vi "Subscribe to Request-Reply.vi"(8 "error in (no error)":errorcluster, 11 "Request-Reply Reference in":refnum<data-value>) -> (0 "error out":errorcluster, 3 "Request-Reply Reference out":refnum<data-value>)   [LabVIEW 2018, in "Scripting.lvlib"]
uses:
  Scripting.lvlib
  Actor/Stop.ctl
  Actor/Did Stop.ctl
  Actor/Actor.lvclass
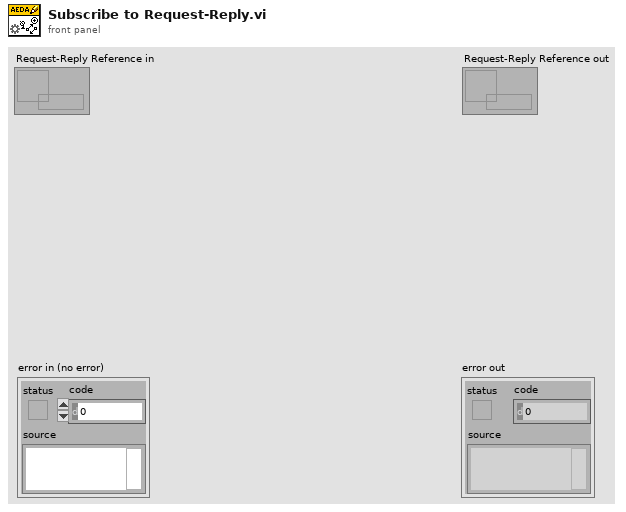
[diagram p1: front panel]
types:
  T1 = typedef "Scripting.lvlib/Actor.lvclass/Stop.ctl" = cluster{"Type":enum16{"Normal", "Emergency"}}
  T2 = cluster{"Stop":refnum<user-event>, "cluster":cluster{"Stopped":refnum<user-event>, "Stop":T1}}
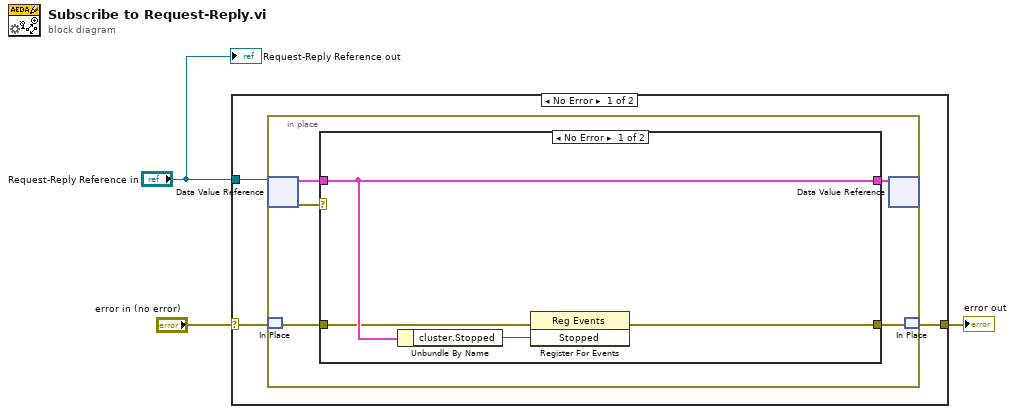
[diagram p0: block diagram]
diagram:
  n1 = case shown="No Error" "error in (no error)" {
    selector: "error in (no error)" -> [w6 w18]
    tunnel: [w5 w18] -> w2
    tunnel: "Request-Reply Reference in" -> [w4 _]
    frame No Error {
      n2 = in-place {
        n3 = in-place-dvr #1(w4) -> (w10:T2, w11:errorcluster)
        n4 = in-place-match #2(w6) -> (w8:errorcluster)
        n5 = case shown="No Error" w11 {
          selector: w11 -> [_ w17]
          tunnel: w10 -> [w15 w16]
          tunnel: [w15 w16] -> w9
          tunnel: w8 -> [w14 _]
          tunnel: [w12 w17] -> w7
          frame No Error {
            n6 = Unbundle By Name(w15) -> ("cluster.Stopped"=w13:refnum<user-event>)
            n7 = register-events(error in=w14, w13) -> (error out=w12:errorcluster)  [unwired: 1 in, 1 out]
          }
          frame Error {
          }
        }
        n8 = in-place-dvr #1(w9) -> ()  [unwired: 2 out]
        n9 = in-place-match #2(w7) -> (w5:errorcluster)
      }
    }
    frame Error {
    }
  }
  "error out" <- w2
  "Request-Reply Reference out" <- "Request-Reply Reference in"
